vi "32-Bit Bidirectional Counter Controller.vi"(8 "Enable":bool, 9 "Direction":bool, 10 "Reset":bool, 11 "Value":u32) -> (3 "Value+":u32)   [LabVIEW 2013]
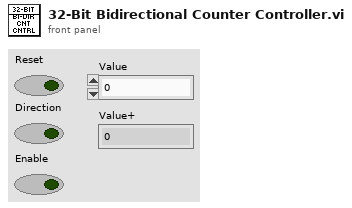
[diagram p1: front panel]
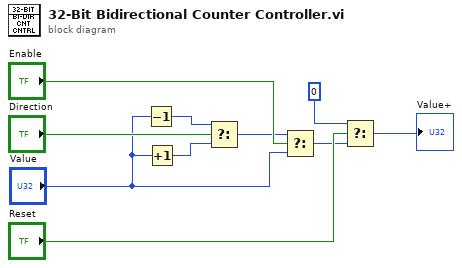
[diagram p0: block diagram]
diagram:
  n1 = Decrement(x="Value") -> (x-1=w6:u32)
  n2 = Increment(x="Value") -> (x+1=w5:u32)
  n3 = Select(t=w6, s="Direction", f=w5) -> (s? t:f=w4:u32)
  n4 = Select(t=w4, s="Enable", f="Value") -> (s? t:f=w2:u32)
  n5 = Select(t=u32 0, s="Reset", f=w2) -> (s? t:f=→"Value+":u32)
